vi "Destroy.vi"(8 "Error In":errorcluster, 11 "reference in":refnum<class "Network Mangement.lvclass">) -> (0 "Error Out":errorcluster, 3 "reference out":refnum<class "Network Mangement.lvclass">)   [LabVIEW 2024, in "CANopen Master.lvlib" / "Network Mangement.lvclass"]
uses:
  Network Mangement.lvclass
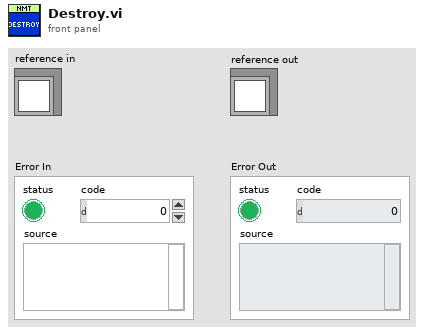
[diagram p1: front panel]
types:
  T1 = typedef "CANopen Master.lvlib/Network Mangement.lvclass/ObjectAttributes.ctl" = cluster{"Nodes":map{u8, u8}, "Heartbeats":map{u8, cluster{"Period":u16, "Timeout":u16, "Last Beat":timestamp}}, "Events":cluster{"Stop Heartbeat Checker":refnum<user-event>, "Heartbeat Timeout":refnum<user-event>, "Heartbeat Checker Error":refnum<user-event>}, "Heartbeat Checker":refnum<vi>}
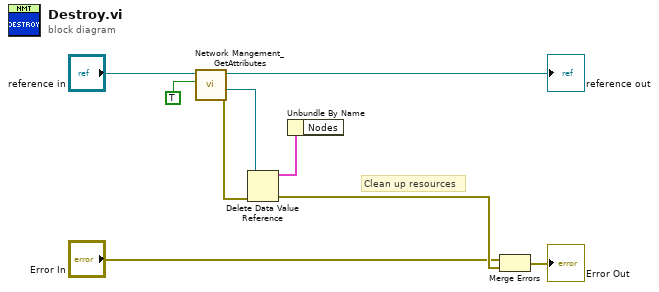
[diagram p0: block diagram]
diagram:
  # "Clean up resources"
  n1 = call "Network Mangement_GetAttributes.vi"("OnlyGetDvrReference(False)"=TRUE, "reference in"="reference in") -> ("Error Out"=w6:errorcluster, "DataRef"=w5:refnum<data-value>, "reference out"=→"reference out":refnum<class "Network Mangement.lvclass">)  [unwired: 6 in, 1 out]
  n2 = Delete Data Value Reference(data value reference=w5, error in=w6) -> (data value=w1:T1, error out=w4:errorcluster)
  n3 = Unbundle By Name(w1) -> ()  [unwired: 1 out]
  n4 = Merge Errors("Error In", w4) -> (→"Error Out":errorcluster)
